vi "Pulse Width Modulation (FPGA).vi"(2 "PWM Period (Ticks)":u32=2000, 3 "PWM Duty Cycle (Ticks)":i32, 6 "Min Period (Ticks)":u32=1000, 7 "Sample Clock Advance (Ticks)":u32=9, 8 "Duty Limit (Ticks)":u32=100, 9 "PID Clock Advance (Ticks)":u32=50, 11 "Rate Limit (Ticks/Cycle)":i32=1000) -> (12 "Actual Duty Cycle (Ticks)":u32, 15 "PWM DO":bool, 16 "PID Clock":bool, 17 "Sample Clock":bool, 18 "Changed?":bool, 19 "Telapsed (Ticks)":u32)   [LabVIEW 2012]
doc: "Generates a digital pulse width modulation (PWM) signal. PWM signals are useful for driving loads such as motors and proportional valves because the average voltage supplied is equal to the PWM duty cycle. The output of this function can be connected to digital output modules. This function is designed for use in LabVIEW FPGA.\n\nOPERATION\nAt the beginning of each cycle the PWM Duty Cycle (Ticks) input is read and the PWM DO digital output is turned on. The digital output is left on for the amount of time specified by the PWM Duty Cycle (Ticks) input. The cycle repeats when the amount of time specified by the PWM Period (Ticks) has elapsed. The FPGA tick counter is used to calculate elapsed time. By default, one tick is equal to 25 nanoseconds (40 MHz), so a PWM Period (Ticks) of 2,000 results in a 20 kHz PWM signal. The PWM Duty Cycle (Ticks) input is a signed integer, but the sign of the value is ignored. Some applications use the sign of the PWM Duty Cycle (Ticks) signal to determine which direction to drive the motor.\n\nUse the rising edge of the PID Clock signal to trigger your FPGA-based current control PID loop execution. The rising edge of the PID Clock signal occurs just before the end of the PWM cycle. The amount of time before the end of the cycle the edge occurs is determined by the PID Clock Advance (Ticks) signal.\n\nUse the rising edge of the Sample Clock signal to trigger your analog input operation to read the motor current for closed loop control. The Sample Clock signal goes TRUE at the mid-point of the PWM DO output and goes FALSE at the beginning of the PWM cycle. For an inductive load, sampling the current at this time gives a rough estimate of the average current. The Sample Clock signal will continue to be generated even if the duty cycle is 0 or 100 percent. In those cases, the rising edge of the Sample Clock signal occurs at the beginning of the PWM cycle. The Sample Clock Advance (Ticks) signal is used to cause the rising edge to occur slightly before the PWM DO mid-point, to compensate for analog input sampling time. For the NI 9505 module, the analog input sampling occurs 9 FPGA clock ticks after the start of the FPGA I/O Node function.\n\nThe Telapsed (Ticks) signal can be used to trigger other operations at particular time in the PWM cycle. For instance, you could use this signal to trigger an analog input operation to occur once per PWM cycle at a programmable time within the PWM cycle. This counter resets back to 0 at the beginning of every PWM cycle.\n\nThe Min Period (Ticks) control is used to limit the PWM Period to prevent switching at frequencies that could damage the output MOSFETs in a digital output device. By default Min Period (Ticks) is set to 1000 ticks, which limits the PWM switching frequency to 40 kHz.\n\nThe Duty Limit (Ticks) control is used to limit the minimum ON and OFF time for the PWM output. If the Duty Cycle is less than the limit, it will be coerced to 0%. If the duty cycle is greater than the Period minus the Duty Limit, the Duty Cycle will be coerced to 100%. Some output devices such as the NI 9505 motor drive module require that the ON and OFF time not be less than a certain limit (2.5 microseconds for the NI 9505). By default Duty Limit (Ticks) is set to 100 ticks, or 2.5 microseconds.\n\nTo obtain the highest timing resolution when using this function in a loop, you can perform digital output I/O operations only when the PWM DO value has changed (rather than on every cycle). To do this, wire the Changed? output to the conditional terminal on a case structure and perform the I/O operation when the case is True. If the duty cycle is 0 or 100%, the Changed? output will strobe true once per PWM cycle at the beginning of the cycle.\n\nThis subVI is reentrant, so you can place multiple instances of the function in a LabVIEW FPGA application and they each will operate independently.\n\nINPUTS\nPWM Period (Ticks)- Total width of the pulse (inverse of the \"PWM Frequency\")\nPWM Duty Cycle (Ticks)- Time for which signal output stays True\nMin Period (Ticks)- The minimum allowed value for the PWM Period\nDuty Limit (Ticks)- The minimum allowed value for the PWM on time and off time\nPID Clock Advance (Ticks)- Determines how many clock ticks before the end of the PWM cycle that the PID Clock rising edge occurs\nSample Clock Advance (Ticks)- Determines how many clock ticks before the mid-point of the PWM digital output that the Sample Clock rising edge occurs \n\nOUTPUTS\nPWM DO- Digital PWM signal that can be connected to a digital output channel I/O node\nPID Clock- clock signal that can be used for synchronizing the execution of a current control PID loop\nSample Clock- clock signal that can be used to trigger an analog input operation to measure the average current in an inductive load\nChanged?- Value is True for one iteration when the PWM DO value has changed, or at the beginning of the PWM cycle if the duty cycle is 0 or 100%\nTelapsed- The amount of time elapsed during the current PWM cycle\n\nSCALING\n\nThe formulas below can be used for scaling from units of Hz, seconds, or percent duty cycle in the real-time host interface application. These formulas assume a 40 MHz (40,000,000 Ticks/sec) FPGA clock rate.\n\nPWM Period (Ticks) = 40,000,000 / PWM Period (Hz)\nPWM Period (Ticks) = 40,000,000 * PWM Period (sec)\nPWM Duty Cycle (Ticks) = PWM Period (Ticks) * PWM Duty Cycle (%) / 100\nPWM Duty Cycle (Ticks) = 40,000,000 * PWM Duty Cycle (sec)"
uses:
  <vilib>/Platform/TimedLoop/XDataNode/timing_clust.ctl
  <vilib>/Platform/TimedLoop/XDataNode/nitl_modes.ctl
  <vilib>/Platform/TimedLoop/XDataNode/wakeup.ctl
  Instance           5 37Saved   Pulse Width Modulation (FPGA) .vi
  <vilib>/Platform/TimedLoop/XDataNode/XDataNode.xnode
  <vilib>/rvi/Arithmetic/AddSubMult/XNode/nirviSatArithmetic.xnode
  <vilib>/Platform/TimedLoop/XDataNode/XDNodeRunTimeDep.lvlib
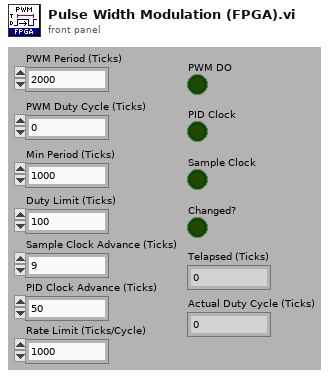
[diagram p1: front panel]
types:
  T1 = typedef "XDNodeRunTimeDep.lvlib/timing_clust.ctl" = cluster{"Expected End [f-1]":u64, "Actual End [f-1]":u64, "Finished Late? [f-1]":bool, "Expected End [i-1]":u64, "Actual End [i-1]":u64, "Finished Late? [i-1]":bool, "Expected Start [i]":u64, "Actual Start [i]":u64, "Expected Start [f]":u64, "Actual Start [f]":u64, "Source Name":string, "Structure Name":string, "Period":i64, "Deadline":i64, "Offset":i64, "Start":i64, "Priority":i32, "Timeout":i32, "Mode":T2, "Wakeup Reason":T3, "Error":errorcluster, "Source Type":string, "Secondary Source Type":string, "Global End Time":u64, "Global Start Time":u64, "Frame Duration":u64, "Iteration Duration":u64, "Assigned CPU":i32, "I/O Scan Engine Mode":u32}
  T2 = typedef "XDNodeRunTimeDep.lvlib/nitl_modes.ctl" = enum32{"No Change", "Process missed periods, maintain original phase", "Discard missed periods, maintain original phase", "Process missed periods, ignore original phase", "Discard missed periods, ignore original phase"}
  T3 = typedef "XDNodeRunTimeDep.lvlib/wakeup.ctl" = enum32{"Normal", "Aborted", "Asynchronous wakeup", "Timing source error", "Timed loop error", "Timeout"}
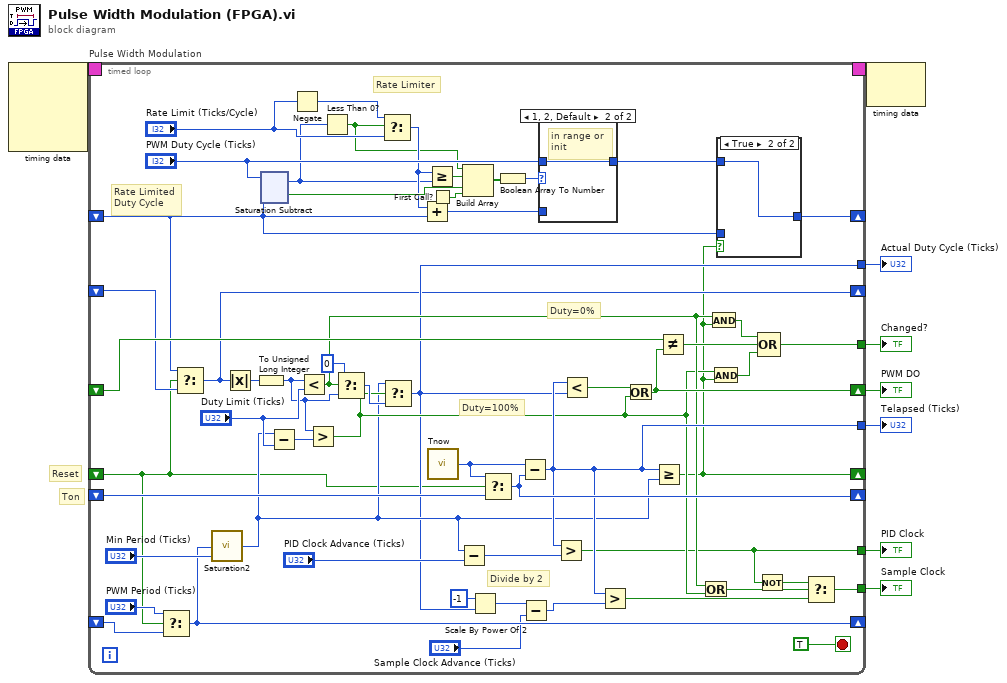
[diagram p0: block diagram]
diagram:
  # "Reset"
  # "Ton"
  n1 = node-c288() -> (w4:T1)  [unwired: 4 in]
  n2 = timed-loop "Pulse Width Modulation" {
    shift-right: [w61] -> _
    shift-left: _ -> [w62]
    shift-right: [w15] -> _
    shift-left: _ -> [w23]
    tunnel: [w45] -> w8
    tunnel: [w40] -> w7
    shift-right: [w52] -> w6
    shift-left: _ -> [w60]
    tunnel: [w56] -> w5
    timing: w4 -> [_]
    timing-out: [_] -> w3
    tunnel: [w38] -> w2
    shift-right: [w35] -> _
    shift-left: _ -> [w36]
    shift-right: [w14] -> _
    shift-left: _ -> [w12]
    tunnel: [w28] -> w1
    shift-right: [w27] -> _
    shift-left: _ -> [w26]
    stop <- TRUE stop-if-true
    # "Rate Limiter"
    # "Rate Limited\nDuty Cycle"
    # "Duty=100%"
    # "Duty=0%"
    # "Divide by 2"
    n3 = Select(t="PWM Period (Ticks)", s=w23, f=w36) -> (s? t:f=w35:u32)
    n4 = Select(t=w12, s=w23, f=w26) -> (s? t:f=w27:i32)
    n5 = call "Saturation2"("input"=w35, "lower limit"="Min Period (Ticks)") -> ("output"=w29:u32)  [unwired: 7 in]
    n6 = Absolute Value(x=w27) -> (abs(x)=w55:i32)
    n7 = To Unsigned Long Integer(number=w55) -> (unsigned 32bit integer=w49:u32)
    n8 = xnode ("Saturation Subtract")("x"="PWM Duty Cycle (Ticks)", "y"=w12) -> ("x-y"=w9:i32, "overflow"=w21:bool)
    n9 = Subtract(x=w29, y="Duty Limit (Ticks)") -> (x-y=w47:u32)
    n10 = Negate(x="Rate Limit (Ticks/Cycle)") -> (-x=w22:i32)
    n11 = Less?(x=w49, y="Duty Limit (Ticks)") -> (x < y?=w44:bool)
    n12 = Greater?(x=w49, y=w47) -> (0:w43:bool)
    n13 = Less Than 0?(x=w9) -> (x < 0?=w10:bool)
    n14 = Select(t=u32 0, s=w44, f=w49) -> (s? t:f=w48:u32)
    n15 = Select(t=w22, s=w10, f="Rate Limit (Ticks/Cycle)") -> (s? t:f=w19:i32)
    n16 = Select(t=w29, s=w43, f=w48) -> (s? t:f=w28:u32)
    n17 = Add(x=w19, y=w12) -> (x+y=w20:i32)
    n18 = Greater Or Equal?(x=w19, y=w9) -> (x >= y?=w16:bool)
    n19 = First Call?() -> (First Call?: T/F=w11:bool)
    n20 = call "Tnow"() -> ("Tick Count(Ticks)"=w63:u32)
    n21 = Subtract(x=w29, y="PID Clock Advance (Ticks)") -> (x-y=w31:u32)
    n22 = Build Array(w10, w16, w21, w11) -> (w17:bool[])
    n23 = Scale By Power Of 2(n=i8 -1, x=w28) -> (x*2^n=w34:u32)
    n24 = Select(t=w63, s=w23, f=w62) -> (s? t:f=w61:u32)
    n25 = Boolean Array To Number(Boolean array=w17) -> (number=w18:u8)
    n26 = Subtract(x=w63, y=w61) -> (x-y=w45:u32)
    n27 = Subtract(x=w34, y="Sample Clock Advance (Ticks)") -> (x-y=w33:u32)
    n28 = case shown="1, 2, Default" w18 {
      tunnel: w20 -> [w85 _]
      tunnel: "PWM Duty Cycle (Ticks)" -> [_ w86]
      tunnel: [w85 w86] -> w13
      frame 0, 3..7 {
        # "out of range"
      }
      frame 1, 2, Default {
        # "in range or \ninit"
      }
    }
    n29 = Greater?(x=w45, y=w31) -> (0:w40:bool)
    n30 = Less?(x=w45, y=w28) -> (x < y?=w58:bool)
    n31 = Greater?(x=w45, y=w33) -> (0:w39:bool)
    n32 = Or(x=w58, y=w43) -> (x .or. y?=w52:bool)
    n33 = Greater Or Equal?(x=w45, y=w29) -> (x >= y?=w15:bool)
    n34 = Not Equal?(x=w60, y=w52) -> (x != y?=w59:bool)
    n35 = Or(x=w44, y=w43) -> (x .or. y?=w42:bool)
    n36 = And(x=w44, y=w15) -> (x .and. y?=w54:bool)
    n37 = And(x=w43, y=w15) -> (x .and. y?=w53:bool)
    n38 = case shown="True" w15 {
      tunnel: [w83 w84] -> w14
      tunnel: w13 -> [_ w84]
      tunnel: w12 -> [w83 _]
      frame False {
      }
      frame True {
      }
    }
    n39 = Not(x=w40) -> (.not. x?=w41:bool)
    n40 = Compound Arithmetic op=OR(w54, w59, w53) -> (w56:bool)
    n41 = Select(t=w41, s=w42, f=w39) -> (s? t:f=w38:bool)
  }
  "Telapsed (Ticks)" <- w8
  "PID Clock" <- w7
  "PWM DO" <- w6
  "Changed?" <- w5
  "Sample Clock" <- w2
  "Actual Duty Cycle (Ticks)" <- w1
  n42 = node-c288(w3) -> ()  [unwired: 1 out]
